vi "Test wait vs wait on notify.vi"() -> ()   [LabVIEW 2014]
panel:
  out "x-y 2":dbl format="%#.6f"
  out "x-y":dbl format="%#.6f"
  out "Waveform Chart 4":dbl(graph)
  out "Waveform Chart 3":dbl(graph)
  in  "Boolean":bool
  out "Waveform Chart 2":dbl(graph)
  out "Waveform Chart":dbl(graph)
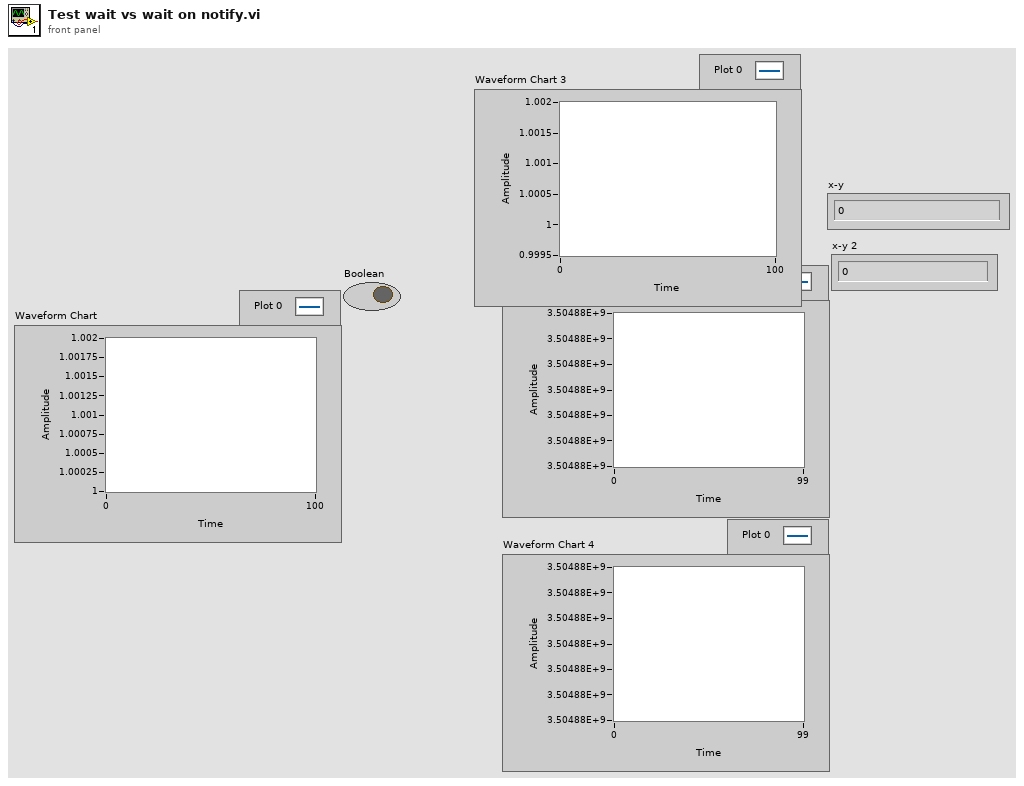
[diagram p1: front panel]
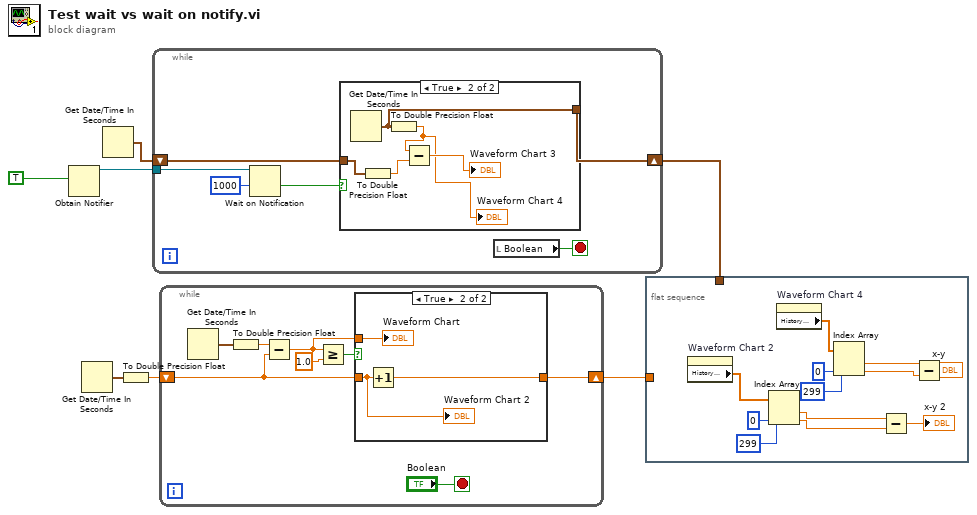
[diagram p0: block diagram]
diagram:
  n1 = Obtain Notifier(notification data type=TRUE) -> (notifier out=w4:refnum<notifier>)  [unwired: 3 in, 2 out]
  n2 = Get Date/Time In Seconds() -> (seconds since 1Jan1904=w7:timestamp)
  n3 = Get Date/Time In Seconds() -> (seconds since 1Jan1904=w3:timestamp)
  n4 = To Double Precision Float(number=w7) -> (double precision float=w6:dbl)
  n5 = while {
    tunnel: w4 -> [w12]
    shift-right: [w8] -> w2
    shift-left: w3 -> [w9]
    stop <- w13 stop-if-true
    n6 = Wait on Notification(notifier=w12, timeout in ms (-1)=1000) -> (timed out?=w10:bool)  [unwired: 2 in, 3 out]
    n7 = case shown="True" w10 {
      tunnel: w9 -> [w14 w18]
      tunnel: [w14 w17] -> w8
      frame False {
      }
      frame True {
        n8 = Get Date/Time In Seconds() -> (seconds since 1Jan1904=w17:timestamp)
        n9 = To Double Precision Float(number=w18) -> (double precision float=w19:dbl)
        n10 = To Double Precision Float(number=w17) -> (double precision float=w15:dbl)
        "Waveform Chart 4" <- w15
        n11 = Subtract(x=w15, y=w19) -> (x-y=→"Waveform Chart 3":dbl)
      }
    }
    n12 = local read "Boolean"() -> (w13:bool)
  }
  n13 = while {
    shift-right: [w22] -> w1
    shift-left: w6 -> [w23]
    stop <- "Boolean" stop-if-true
    n14 = Get Date/Time In Seconds() -> (seconds since 1Jan1904=w27:timestamp)
    n15 = To Double Precision Float(number=w27) -> (double precision float=w26:dbl)
    n16 = Subtract(x=w26, y=w23) -> (x-y=w21:dbl)
    n17 = Greater Or Equal?(x=w21, y=1.0) -> (x >= y?=w24:bool)
    n18 = case shown="True" w24 {
      tunnel: w23 -> [w28 w29]
      tunnel: [w28 w31] -> w22
      tunnel: w21 -> [_ w30]
      frame False {
      }
      frame True {
        n19 = Increment(x=w29) -> (x+1=w31:dbl)
        "Waveform Chart" <- w30
        "Waveform Chart 2" <- w29
      }
    }
  }
  n20 = flat-sequence {
    tunnel: w2 -> [_]
    tunnel: w1 -> [_]
    frame #0 {
      n21 = property on="Waveform Chart 2" class="WFChart (strict)"() -> ("History Data"=w43:dbl[])  [unwired: 2 in, 2 out]
      n22 = Index Array(array=w43, index #1=299 ("index"), index #2=0 ("index")) -> (element #1=w33:dbl, element #2=w32:dbl)
      n23 = property on="Waveform Chart 4" class="WFChart (strict)"() -> ("History Data"=w38:dbl[])  [unwired: 2 in, 2 out]
      n24 = Index Array(array=w38, index #1=299 ("index"), index #2=0 ("index")) -> (element #1=w34:dbl, element #2=w35:dbl)
      n25 = Subtract(x=w33, y=w32) -> (x-y=→"x-y 2":dbl)
      n26 = Subtract(x=w34, y=w35) -> (x-y=→"x-y":dbl)
    }
  }
